vi "Get System Channels Info.vi"(8 "error in (no error)":errorcluster, 11 "Item Ref in":T1 format="%.0x") -> (0 "error out":errorcluster, 2 "System Channel Refs":T1[](array[typedef]) format="%.0x", 3 "Item Ref out":T1 format="%.0x")   [LabVIEW 2019, in "Telemetry Engine.lvlib"]
uses:
  Telemetry Engine.lvlib
  <vilib>/NI VeriStand/Custom Device API/Custom Device Item Ref.ctl
  <vilib>/NI VeriStand/Custom Device Tools/Custom Device Utility Library/Custom Device Utility Library.lvlib
  <vilib>/NI VeriStand/Custom Device API/Custom Device API.lvlib
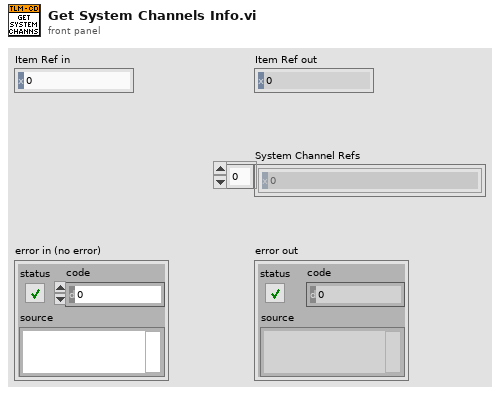
[diagram p1: front panel]
types:
  T1 = typedef "Custom Device API.lvlib/Custom Device Item Ref.ctl" = u64
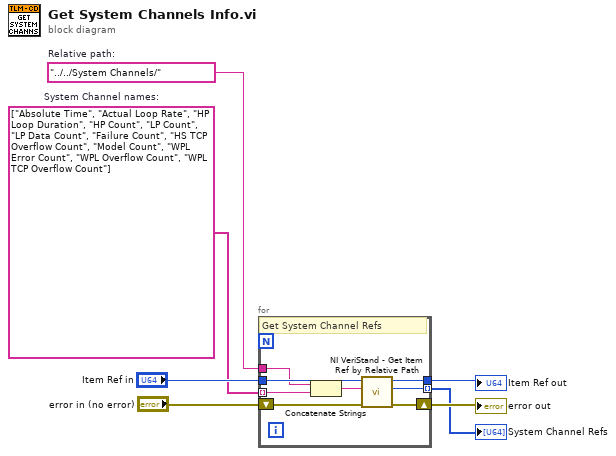
[diagram p0: block diagram]
diagram:
  w1 = "../../System Channels/"  # Relative path:
  w2 = string[] ["Absolute Time", "Actual Loop Rate", "HP Loop Duration", "HP Count", "LP Count", "LP Data Count", "Failure Count", "HS TCP Overflow Count", "Model Count", "WPL Error Count", "WPL Overflow Count", "WPL TCP Overflow Count"]  # System Channel names:
  n1 = for {
    tunnel: "Item Ref in" -> [w15]
    shift-right: [w9] -> w6
    shift-left: "error in (no error)" -> [w14]
    tunnel: [w13] -> w5
    tunnel: [w8] -> w4 mode=indexing
    tunnel: w2 -> [w12] mode=indexing
    tunnel: w1 -> [w11]
    # "Get System Channel Refs"
    n2 = Concatenate Strings(w11, w12) -> (w10:string)
    n3 = call <vilib>:"NI VeriStand - Get Item Ref by Relative Path.vi"("error in"=w14, "Relative Item Path"=w10, "Section Ref in"=w15) -> ("error out"=w9:errorcluster, "Item Ref"=w8:T1, "Section Ref out"=w13:T1)  [unwired: 5 in, 1 out]
  }
  "error out" <- w6
  "Item Ref out" <- w5
  "System Channel Refs" <- w4
